vi "Mask sub VI.vi"(0 "Image In":T4, 1 "Mask&Edge ROI param":T1, 11 "error out":errorcluster) -> (4 "Gray Level Image out":T4, 6 "Binary Image out":T4, 10 "ROI Descriptor":T3 {"Contours"."Type" items=["No Selection", "Point", "Line", "Rectangle", "Oval", "Polygon", "Freehand Region", "Annulus", "Unused2", "Unused3", "Broken Line", "Freehand Line", "Rotated Rectangle"]}, 13 "Centroid of blob":dbl[][](array[numeric]) format="%.2f", 14 "Rectangle for overlay":T2, 15 "error out":errorcluster)   [LabVIEW 2019, in "Algorithm.lvclass"]
uses:
  FrameworkOverrides/Algorithm.lvclass
  <vilib>/vision/NI_Vision_Development_Module.lvlib
  <vilib>/vision/Image Controls.llb/IMAQ Image.ctl
panel:
  # "INPUTS"
  # "OUTPUTS"
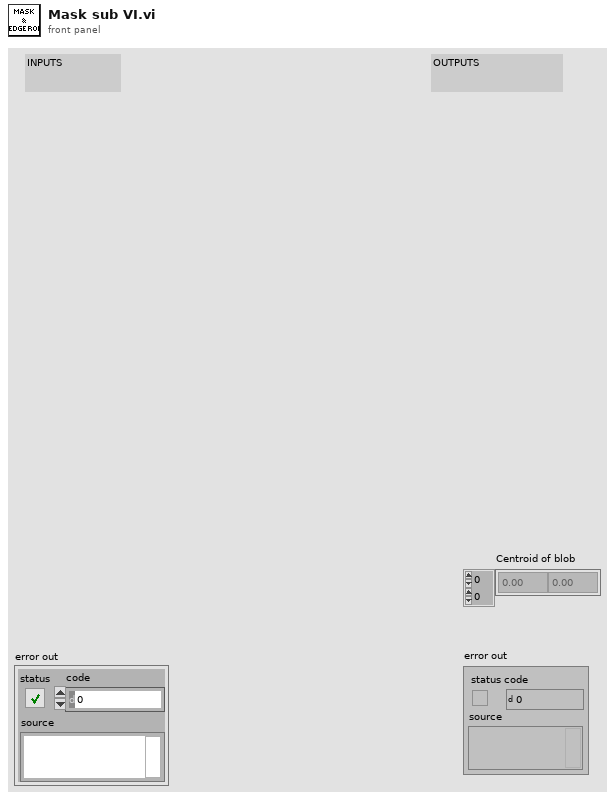
[diagram p1: front panel]
types:
  T1 = cluster{"Lower thresh":sgl, "Upper thresh":sgl, "Xoffset":sgl, "Y offset":sgl}
  T2 = cluster{"Left":i32, "Top":i32, "Right":i32, "Bottom":i32}
  T3 = typedef "ROI Descriptor" = cluster{"Global Rectangle":i32[], "Contours":cluster{"ID":enum32{"External", "Internal"}, "Type":u32, "Coordinates":i32[]}[]}
  T4 = typedef "IMAQ Image.ctl" = refnum<image>
  T5 = typedef "IMAQ Rectangle" = cluster{"Left":i32, "Top":i32, "Right":i32, "Bottom":i32, "Rotation":dbl}
  T6 = typedef "Particle Parameters" = i32
  T7 = cluster{"Measurement Parameter":T6, "Range Lower Value":dbl, "Range Upper Value":dbl, "Range":bool, "Measurement Type":bool}[]
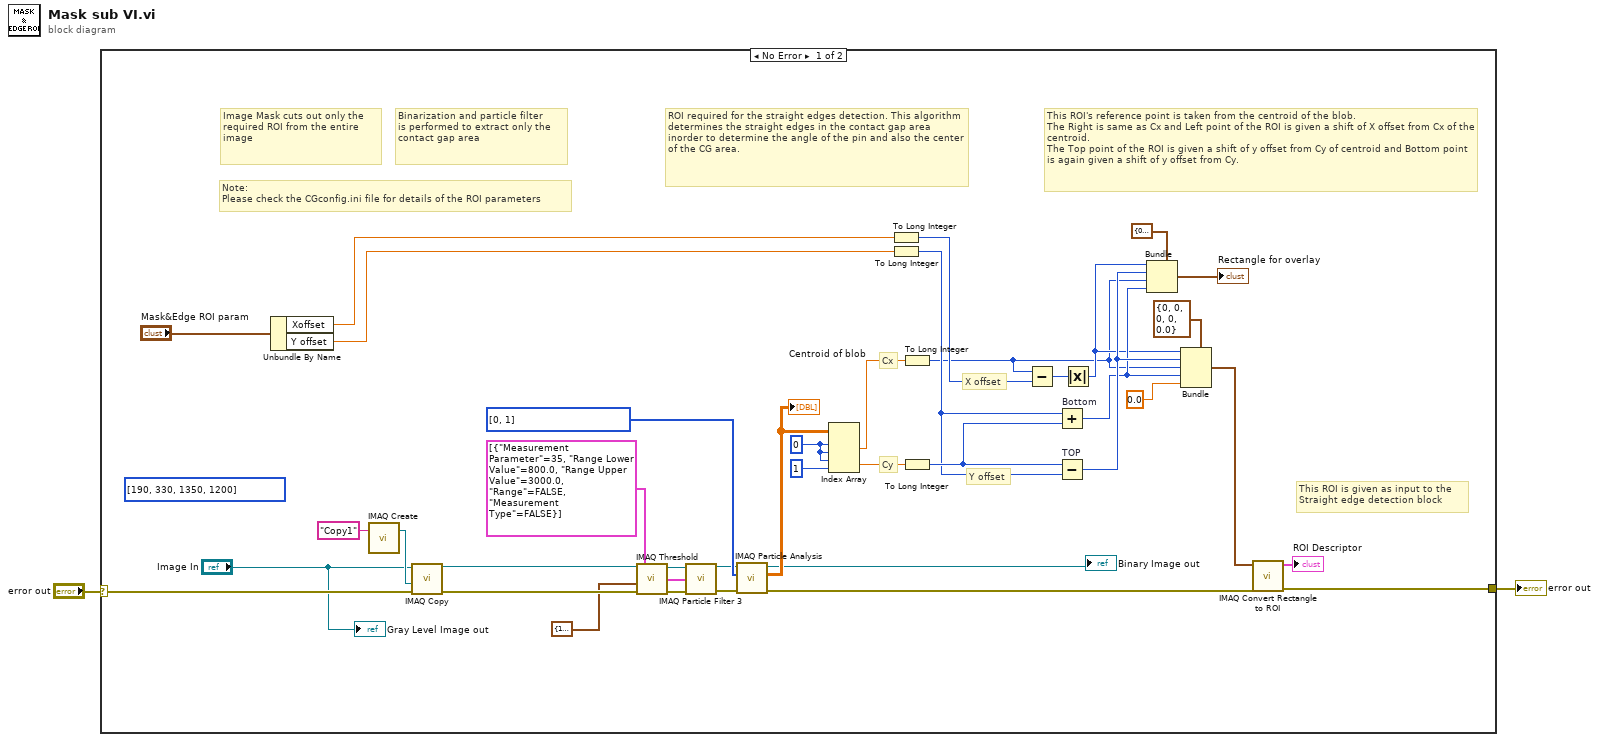
[diagram p0: block diagram]
diagram:
  n1 = case shown="No Error" "error out" {
    selector: "error out" -> [w4 w41]
    tunnel: [w27 w41] -> w2
    frame No Error {
      (unwired) i32[] [190, 330, 1350, 1200] ("Global Rectangle")
      w36 = 0 ("index (row)")
      w39 = T6[] [0, 1] items=["Center of Mass X", "Center of Mass Y", "First Pixel X", "First Pixel Y", "Bounding Rect Left", "Bounding Rect Top", "Bounding Rect Right", "Bounding Rect Bottom", "Max Feret Diameter Start X", "Max Feret Diameter Start Y", "Max Feret Diameter End X", "Max Feret Diameter End Y", "Max Horiz. Segment Length Left", "Max Horiz. Segment Length Right", "Max Horiz. Segment Length Row", "-", "Bounding Rect Width", "Bounding Rect Height", "Bounding Rect Diagonal", "Perimeter", "Convex Hull Perimeter", "Holes' Perimeter", "Max Feret Diameter", "Equivalent Ellipse Major Axis", "Equivalent Ellipse Minor Axis", "Equivalent Ellipse Minor Axis (Feret)", "Equivalent Rect Long Side", "Equivalent Rect Short Side", "Equivalent Rect Diagonal", "Equivalent Rect Short Side (Feret)", "Average Horiz. Segment Length", "Average Vert. Segment Length", "Hydraulic Radius", "Waddel Disk Diameter", "-", "Area", "Holes' Area", "Particle & Holes' Area", "Convex Hull Area", "Image Area", "-", "Number of Holes", "Number of Horiz. Segments", "Number of Vert. Segments", "-", "Orientation", "Max Feret Diameter Orientation", "-", "% Area/Image Area", "% Area/(Particle & Holes' Area)", "Ratio of Equivalent Ellipse Axes", "Ratio of Equivalent Rect Sides", "-", "Elongation Factor", "Compactness Factor", "Heywood Circularity Factor", "Type Factor", "-", "Sum X", "Sum Y", "Sum XX", "Sum XY", "Sum YY", "Sum XXX", "Sum XXY", "Sum XYY", "Sum YYY", "-", "Moment of Inertia XX", "Moment of Inertia XY", "Moment of Inertia YY", "Moment of Inertia XXX", "Moment of Inertia XXY", "Moment of Inertia XYY", "Moment of Inertia YYY", "Norm. Moment of Inertia XX", "Norm. Moment of Inertia XY", "Norm. Moment of Inertia YY", "Norm. Moment of Inertia XXX", "Norm. Moment of Inertia XXY", "Norm. Moment of Inertia XYY", "Norm. Moment of Inertia YYY", "Hu Moment 1", "Hu Moment 2", "Hu Moment 3", "Hu Moment 4", "Hu Moment 5", "Hu Moment 6", "Hu Moment 7"] ("Pixel Measurements")
      # "X offset"
      # "Note:\nPlease check the CGconfig.ini file for details of the ROI parameters"
      # "Cy"
      # "Cx"
      # "Y offset"
      # "This ROI's reference point is taken from the centroid of the blob.\nThe Right is same as Cx and Left point of the ROI is given a shift of X offset from Cx of the centroid.\nThe Top point of the ROI is given a shift of y offset from Cy of centroid and Bottom point is again given a shift of y offset from Cy."
      # "This ROI is given as input to the \nStraight edge detection block"
      # "Binarization and particle filter\nis performed to extract only the \ncontact gap area"
      # "Image Mask cuts out only the required ROI from the entire image"
      # "ROI required for the straight edges detection. This algorithm determines the straight edges in the contact gap area inorder to determine the angle of the pin and also the center of the CG area."
      n2 = Unbundle By Name("Mask&Edge ROI param") -> ("Xoffset"=w14:sgl, "Y offset"=w13:sgl)
      n3 = call "IMAQ Create"("Image Name"="Copy1") -> ("New Image"=w33:T4)  [unwired: 4 in, 1 out]
      n4 = call "IMAQ Copy"("error in (no error)"=w4, "Image Dst"=w33, "Image Src"="Image In") -> ("error out"=w31:errorcluster, "Image Dst Out"=w32:T4)  [unwired: 3 in]
      n5 = call "IMAQ Threshold"("error in (no error)"=w31, "Range"=cluster{"Lower value":sgl, "Upper value":sgl} {"Lower value"=100.0, "Upper value"=255.0}, "Image Src"=w32) -> ("error out"=w18:errorcluster, "Image Dst Out"=w19:T4)  [unwired: 7 in]
      n6 = call "IMAQ Particle Filter 3"("Image Src"=w19, "Selection Values"=T7 [{"Measurement Parameter"=35, "Range Lower Value"=800.0, "Range Upper Value"=3000.0, "Range"=FALSE, "Measurement Type"=FALSE}], "error in (no error)"=w18) -> ("Image Dst Out"=w17:T4, "error out"=w16:errorcluster)  [unwired: 10 in, 1 out]
      n7 = call "IMAQ Particle Analysis"("error in (no error)"=w16, "Pixel Measurements"=w39, "Image"=w17) -> ("error out"=w29:errorcluster, "Particle Measurements (Pixels)"=w38:dbl[][], "Image Out (duplicate)"=→"Binary Image out":T4)  [unwired: 3 in, 3 out]
      "Centroid of blob" <- w38
      n8 = Index Array(array=w38, index (row) #1=w36, index (col) #1=w36, index (row) #2=w36, index (col) #2=1 ("index (row)")) -> (element #1=w25:dbl, element #2=w24:dbl)
      n9 = To Long Integer(number=w14) -> (32bit integer=w12:i32)
      n10 = To Long Integer(number=w13) -> (32bit integer=w9:i32)
      n11 = To Long Integer(number=w25) -> (32bit integer=w6:i32)
      n12 = To Long Integer(number=w24) -> (32bit integer=w10:i32)
      n13 = Subtract(x=w6, y=w12) -> (x-y=w8:i32)
      n14 = Add "Bottom"(x=w9, y=w10) -> (x+y=w11:i32)
      n15 = Subtract "TOP"(x=w10, y=w9) -> (x-y=w28:i32)
      n16 = Absolute Value(x=w8) -> (abs(x)=w7:i32)
      n17 = Bundle(cluster=T2 {"Left"=0, "Top"=0, "Right"=0, "Bottom"=0}, "Left"=w7, "Top"=w28, "Right"=w6, "Bottom"=w11) -> (→"Rectangle for overlay":T2)
      n18 = Bundle(cluster=T5 {"Left"=0, "Top"=0, "Right"=0, "Bottom"=0, "Rotation"=0.0} ("Rectangle"), "Left"=w7, "Top"=w28, "Right"=w6, "Bottom"=w11, "Rotation"=0.0) -> (w21:T5)
      n19 = call "IMAQ Convert Rectangle to ROI"("error in (no error)"=w29, "Rectangle"=w21) -> ("error out"=w27:errorcluster, "ROI Descriptor"=→"ROI Descriptor":T3)  [unwired: 7 in]
      "Gray Level Image out" <- "Image In"
    }
    frame Error {
    }
  }
  "error out" <- w2
